vi "refresh source enum.vi"   [LabVIEW 2017]
doc: "SciScan 1.2 160622"
uses:
  Custom Control and Typedefs/ChannelSelector_for_PosSave.ctl
  GFG/GFGfpRefGet.vi
  GFG/GFG library.lvlib
types:
  T1 = typedef "ChannelSelector_for_PosSave.ctl" = enum16{"Channel 1", "Channel 2", "Channel 3", "Channel 4"}
  T2 = cluster{"WaveformChartRef":refnum<vi>, "DigitalRef":refnum<vi>, "ArrayRef":refnum<vi>, "TabControlRef":refnum<vi>, "EnumRef":refnum<vi>, "RingRef":refnum<vi>, "BooleanRef":refnum<vi>, "KnobRef":refnum<vi>, "SlideRef":refnum<vi>, "PathRef":refnum<vi>, "StringRef":refnum<vi>, "ComboBox":refnum<vi>, "WaveformGraphRef":refnum<vi>}
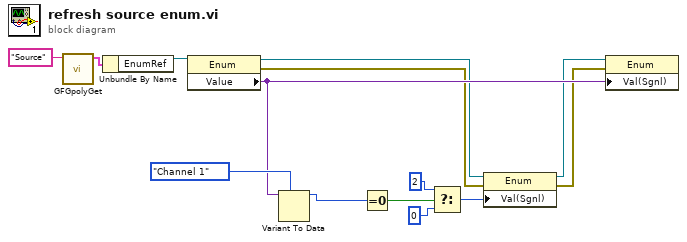
[diagram p0: block diagram]
diagram:
  n1 = call-poly "GFGpolyGet.vi"("Variable Name in"="Source") -> ("output cluster"=w13:T2)  [unwired: 9 in, 1 out]
  n2 = Unbundle By Name(w13) -> ("EnumRef"=w12:refnum<vi>)
  n3 = property class="Enum"(reference=w12) -> (reference out=w4:refnum<vi>, error out=w1:errorcluster, "Value"=w5:variant)  [unwired: 1 in]
  n4 = Variant To Data(type=ChannelSelector_for_PosSave."Channel 1" ("Source"), Variant=w5) -> (data=w10:T1)  [unwired: 1 in, 1 out]
  n5 = Equal To 0?(x=w10) -> (x = 0?=w9:bool)
  n6 = Select(t=2, s=w9, f=0) -> (s? t:f=w6:i32)
  n7 = property class="Enum"(reference=w4, error in=w1, "Val(Sgnl)"=w6) -> (reference out=w3:refnum<vi>, error out=w2:errorcluster)
  n8 = property class="Enum"(reference=w3, error in=w2, "Val(Sgnl)"=w5) -> ()  [unwired: 2 out]
